vi "ArmControlCalibrate.vi"() -> ()   [LabVIEW 2014]
uses:
  <vilib>/Rock Robotics/WPI/CAN/TalonSRX/WPI_CANTalonSRX_APIFeedbackSelect.ctl
  <vilib>/Rock Robotics/WPI/Joystick/WPI_JoystickDeviceEnum.ctl
  <vilib>/Rock Robotics/WPI/CAN/TalonSRX/WPI_CANTalonSRX_APIControlMode.ctl
  <vilib>/Platform/TimedLoop/XDataNode/timing_clust.ctl
  <vilib>/Platform/TimedLoop/XDataNode/nitl_modes.ctl
  <vilib>/Platform/TimedLoop/XDataNode/wakeup.ctl
  <vilib>/Rock Robotics/WPI/SafetyOutput/WPI_SafetyOutputConfigMenu.ctl
  <vilib>/Rock Robotics/WPI/MotorControl/WPI_MotorControlOpenCANTalonSRX.vi
  Team900-VIs/Logitech/F510/F510-X.vi
  <vilib>/Utility/config.llb/Write Key (Double).vi
  <vilib>/Platform/TimedLoop/XDataNode/XDataNode.xnode
  <vilib>/Platform/TimedLoop/XDataNode/XDNodeRunTimeDep.lvlib
  <vilib>/Utility/config.llb/NI_LVConfig.lvlib
panel:
  in  "Motor to set offset":enum16{"Pivot", "Wrist", "Claw"}(ring)
  in  "Set":bool
  in  "stop":bool
  in  "Mode":enum32{"Manual Mode", "PID Tuning"}(tab)
  out "(manual) error out":errorcluster
  out "Sensor Position":dbl
  in  "Control this motor":enum16{"Pivot", "Extension", "Wrist", "Claw"}(ring)
  in  "Max %Vbus":dbl=0.1 format="%#_13g"
  in  "Motor Controller":enum16{"Pivot", "Extension", "Wrist"}(ring)
  in  "PID":cluster{"P":dbl, "I":dbl, "D":dbl}
  out "error out":errorcluster
  in  "Set":bool=TRUE
  in  "Ramp Rate":dbl
  out "Applied Throttle":dbl
  out "Encoder Position":dbl
  out "Analog In":dbl
  out "Sensor Position":dbl
  in  "Enable":bool
  in  "Desired Distance (in) or Angle (rad)":dbl format="%#_13g"
  out "Difference":dbl
  out "Waveform Chart":T1(graph)
  in  "Wrist Offset":dbl format="%#_13g"
  in  "Extension Offset":dbl format="%#_13g"
  in  "Pivot Offset":dbl format="%#_13g"
  in  "Invert Motor (set this before opening)":bool
  # "360 Ticks on extension"
  # "Left Stick controls whatever motor is selected"
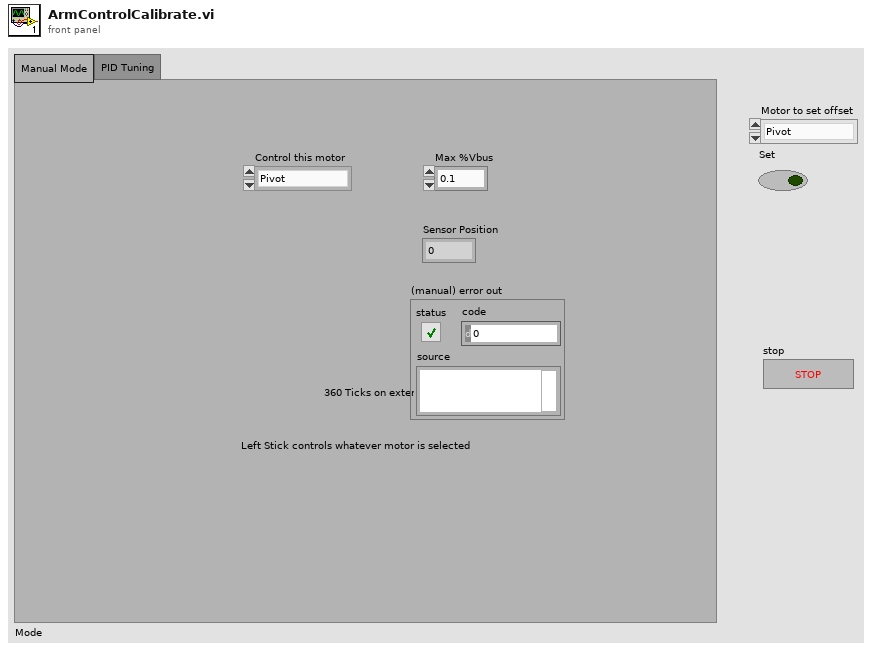
[diagram p1: front panel]
types:
  T1 = cluster{dbl, "Desired Distance (in) or Angle (rad)":dbl}
  T2 = typedef "NI_LVConfig.lvlib/Config Data RefNum.ctl" = refnum<k1>
  T3 = typedef "WPI_JoystickDeviceEnum.ctl" = enum16{"USB 0", "USB 1", "USB 2", "USB 3", "USB 4", "USB 5"}
  T4 = typedef "WPI_CANTalonSRX_APIControlMode.ctl" = enum8{"Percent VBus", "Speed", "Position", "Slave", "Unchanged / Invalid"}
  T5 = typedef "WPI_SafetyOutputConfigMenu.ctl" = enum16{"Enable", "Disable"}
  T6 = typedef "WPI_CANTalonSRX_APIFeedbackSelect.ctl" = enum16{"Digital Quadrature Encoder", "Analog Potentiometer", "Analog Encoder"}
  T7 = typedef "XDNodeRunTimeDep.lvlib/timing_clust.ctl" = cluster{"Expected End [f-1]":u64, "Actual End [f-1]":u64, "Finished Late? [f-1]":bool, "Expected End [i-1]":u64, "Actual End [i-1]":u64, "Finished Late? [i-1]":bool, "Expected Start [i]":u64, "Actual Start [i]":u64, "Expected Start [f]":u64, "Actual Start [f]":u64, "Source Name":string, "Structure Name":string, "Period":i64, "Deadline":i64, "Offset":i64, "Start":i64, "Priority":i32, "Timeout":i32, "Mode":T8, "Wakeup Reason":T9, "Error":errorcluster, "Source Type":string, "Secondary Source Type":string, "Global End Time":u64, "Global Start Time":u64, "Frame Duration":u64, "Iteration Duration":u64, "Assigned CPU":i32, "I/O Scan Engine Mode":u32}
  T8 = typedef "XDNodeRunTimeDep.lvlib/nitl_modes.ctl" = enum32{"No Change", "Process missed periods, maintain original phase", "Discard missed periods, maintain original phase", "Process missed periods, ignore original phase", "Discard missed periods, ignore original phase"}
  T9 = typedef "XDNodeRunTimeDep.lvlib/wakeup.ctl" = enum32{"Normal", "Aborted", "Asynchronous wakeup", "Timing source error", "Timed loop error", "Timeout"}
  T10 = typedef "WPI_MotorControlDeviceRef.ctl" = cluster{"DeviceStatus":errorcluster, "Type":T11, "PWM":cluster{"Controller":T12, "PWM Channel":T13, "DeadBand":T14}, "CAN":cluster{"Device Number":u8, "Control Mode":T15, "Semaphore":T16, "Max Vout":dbl, "TalonSRX Control Mode":T4}, "Invert":bool, "TransformRef":T17, "InvTransformRef":T17}
  T11 = typedef "WPI_MotorControlType.ctl" = enum16{"PWM", "CAN", "CANTalonSRX"}
  T12 = typedef "FPGA_TypedefDigitalModule.ctl" = enum16{"Controller 1"}
  T13 = typedef "FPGA_DIOPWMChannel.ctl" = enum8{"PWM 0", "PWM 1", "PWM 2", "PWM 3", "PWM 4", "PWM 5", "PWM 6", "PWM 7", "PWM 8", "PWM 9", "PWM MXP 0", "PWM MXP 1", "PWM MXP 2", "PWM MXP 3", "PWM MXP 4", "PWM MXP 5", "PWM MXP 6", "PWM MXP 7", "PWM MXP 8", "PWM MXP 9", "Invalid"}
  T14 = typedef "WPI_PWMDeadband.ctl" = cluster{"Name":string, "maxPositivePwm":i32, "minPositivePwm":i32, "centerPwm":i32, "maxNegativePwm":i32, "minNegativePwm":i32, "angularRange":u16}
  T15 = typedef "WPI_CANJaguar_ControlMode.ctl" = enum8{"Percent VBus", "Current", "Speed", "Position", "Voltage"}
  T16 = typedef "Semaphore RefNum" = refnum<k1>
  T17 = typedef "WPI_PWMTransform_ConPane.ctl" = refnum<vi>
  T18 = typedef "WPI_JoystickDevRef.ctl" = cluster{"Device":T3}
  T19 = typedef "WPI_CANTalonSRX_GlobalStatus.ctl" = cluster{"Applied Throttle":dbl, "Module Enabled":bool, "CAN Error":errorcluster, "Closed Loop Error":dbl, "Forward Limit Switch Closed":bool, "Reverse Limit Switch Closed":bool, "Sensor Position":dbl, "Sensor Velocity":dbl, "Current":dbl, "Sticky Fault - Over Temp":bool, "Sticky Fault - Under Voltage":bool, "Sticky Fault - Forward Limit":bool, "Sticky Fault - Reverse Limit":bool, "Sticky Fault - Forward Soft Limit":bool, "Sticky Fault - Reverse Soft Limit":bool, "Brake is Enabled":bool, "Encoder Position":dbl, "Encoder Velocity":dbl, "Encoder Index Count":dbl, "Encoder A Pin State":bool, "Encoder B Pin State":bool, "Encoder Index Pin State":bool, "Analog In":dbl, "Analog In Velocity":dbl, "Temperature (C)":dbl, "Battery Voltage":dbl}
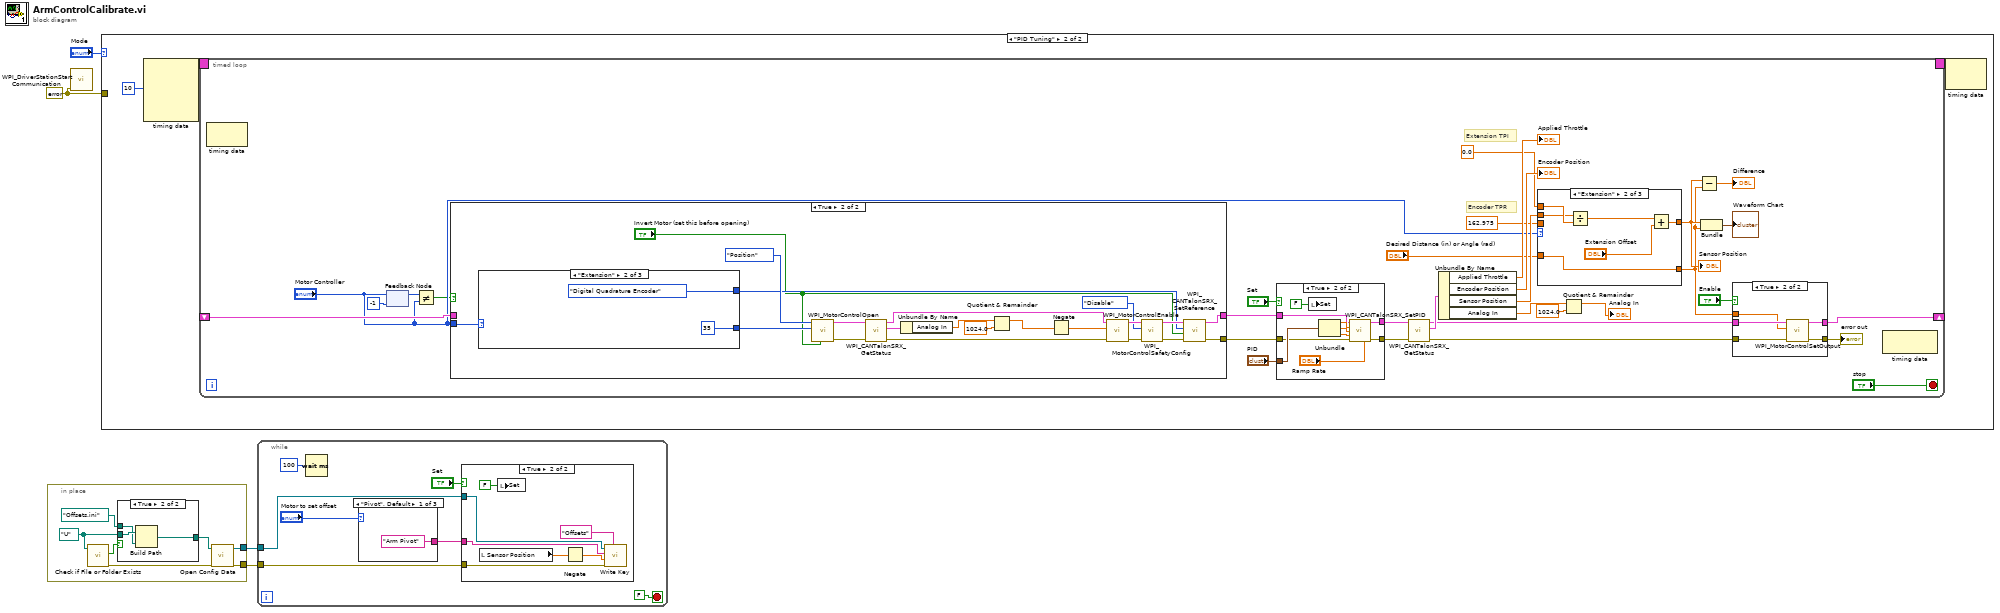
[diagram p0: block diagram]
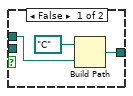
[diagram p2: hidden frame]
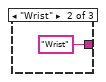
[diagram p3: hidden frame]
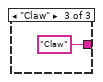
[diagram p4: hidden frame]
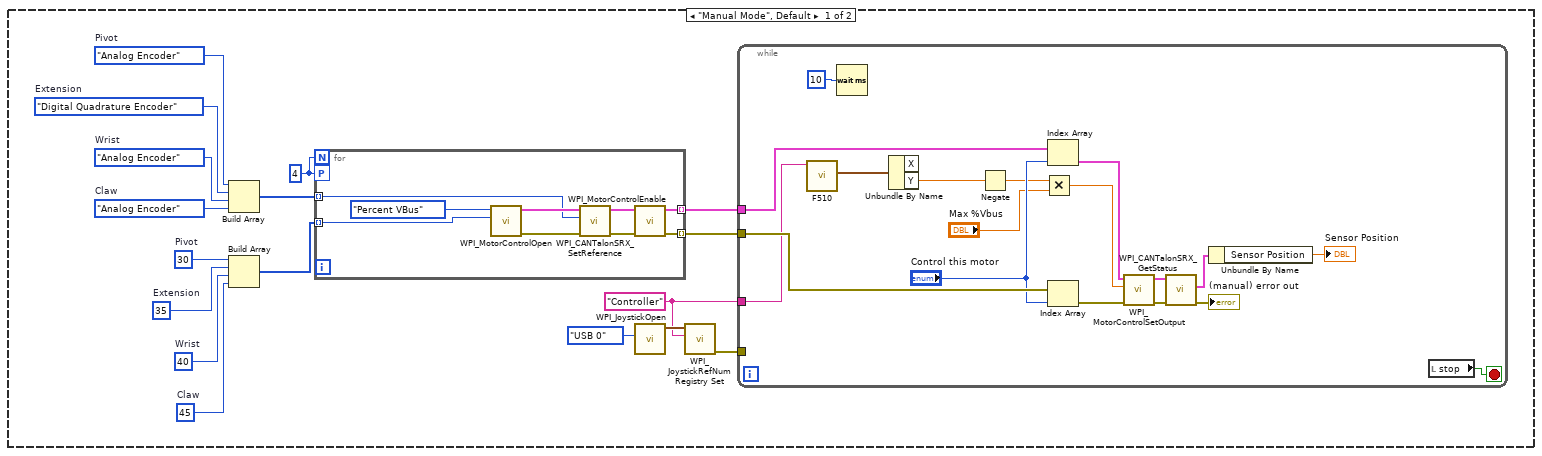
[diagram p6: hidden frame]
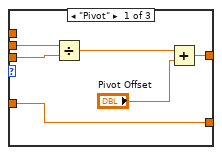
[diagram p7: hidden frame]
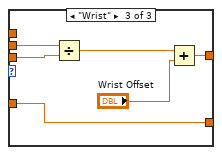
[diagram p8: hidden frame]
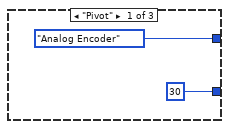
[diagram p10: hidden frame]
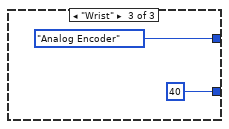
[diagram p11: hidden frame]
diagram:
  w3 = errorcluster {"status"=FALSE, "code"=0, "source"=""} ("error constant")
  n1 = in-place {
    in-place-border: [w10] -> w2
    in-place-border: [w9] -> w1
    w5 = path "U:/" ("base path")
    n2 = call <vilib>:"Check if File or Folder Exists.vi"("path"=w5) -> ("error out"=w11:errorcluster, "file or folder exists?"=w6:bool)  [unwired: 8 in, 1 out]
    n3 = case shown="True" w6 {
      tunnel: path "Offsets.ini" ("default name") -> [w14 w15]
      tunnel: [w13 w16] -> w8
      tunnel: w5 -> [_ w17]
      frame False {
        n4 = Build Path(base path=path "C:/", name or relative path=w14) -> (appended path=w13:path)
      }
      frame True {
        n5 = Build Path(base path=w17, name or relative path=w15) -> (appended path=w16:path)
      }
    }
    n6 = call <vilib>:"Open Config Data.vi"("error in (no error)"=w11, "configuration file path"=w8) -> ("error out"=w10:errorcluster, "refnum"=w9:T2)  [unwired: 1 in, 7 out]
  }
  n7 = call <vilib>:"WPI_DriverStationStart Communication.vi"("error in (no error)"=w3) -> ()  [unwired: 11 in]
  n8 = case shown="\"PID Tuning\"" "Mode" {
    tunnel: w3 -> [_ _]
    frame "Manual Mode", Default {
      w18 = u8 45  # Claw
      w19 = WPI_CANTalonSRX_APIFeedbackSelect."Analog Encoder"  # Claw
      w21 = "Controller" ("refnum name")
      w24 = WPI_CANTalonSRX_APIFeedbackSelect."Analog Encoder"  # Wrist
      w25 = WPI_CANTalonSRX_APIFeedbackSelect."Analog Encoder"  # Pivot
      w26 = WPI_CANTalonSRX_APIFeedbackSelect."Digital Quadrature Encoder"  # Extension
      w30 = u8 40  # Wrist
      w31 = u8 35  # Extension
      w32 = u8 30  # Pivot
      w34 = 4
      n9 = Build Array(w25, w26, w24, w19) -> (w27:T6[])
      n10 = Build Array(w32, w31, w30, w18) -> (w33:u8[])
      n11 = for {
        N: w34 -> [_]
        workers-P: w34 -> [_]
        tunnel: w33 -> [w61] mode=indexing
        tunnel: [w60] -> w29 mode=indexing
        tunnel: [w59] -> w28 mode=indexing
        tunnel: w27 -> [w53] mode=indexing
        n12 = call-poly <vilib>:"WPI_MotorControlOpen.vi"("Device Number"=w61, "Control Mode"=WPI_CANTalonSRX_APIControlMode."Percent VBus") -> ("error out"=w57:errorcluster, "MotorControlDeviceRef"=w56:T10)  [unwired: 8 in]
        n13 = call <vilib>:"WPI_CANTalonSRX_SetReference.vi"("error in (no error)"=w57, "Feedback Reference"=w53, "CAN Talon SRX Ref"=w56) -> ("error out"=w54:errorcluster, "CAN Talon SRX Ref Out"=w55:T10)  [unwired: 7 in]
        n14 = call <vilib>:"WPI_MotorControlEnable.vi"("error in (no error)"=w54, "CAN Jaguar Ref"=w55) -> ("error out"=w59:errorcluster, "CAN Jaguar Ref Out"=w60:T10)  [unwired: 8 in]
      }
      n15 = call <vilib>:"WPI_JoystickOpen.vi"("JoystickDevice"=WPI_JoystickDeviceEnum."USB 0") -> ("JoystickDevRef"=w23:T18)  [unwired: 10 in]
      n16 = call <vilib>:"WPI_JoystickRefNum Registry Set.vi"("refnum name"=w21, "JoystickDevRef"=w23) -> ("error out"=w20:errorcluster)  [unwired: 8 in, 1 out]
      n17 = while {
        tunnel: w29 -> [w51]
        tunnel: w28 -> [w50]
        tunnel: w21 -> [w48]
        tunnel: w20 -> [_]
        stop <- w41 stop-if-true
        n18 = call-poly "F510.vi"("refnum name"=w48) -> ("Left Stick"=w45:cluster{"X":dbl, "Y":dbl})  [unwired: 4 in, 6 out]
        n19 = Wait (ms)(milliseconds to wait=u32 10) -> ()  [unwired: 1 out]
        n20 = Unbundle By Name(w45) -> ("Y"=w44:dbl)  [unwired: 1 out]
        n21 = Negate(x=w44) -> (-x=w35:dbl)
        n22 = Multiply(x=w35, y="Max %Vbus") -> (x*y=w42:dbl)
        n23 = Index Array(array=w51, index="Control this motor") -> (element=w37:T10)
        n24 = Index Array(array=w50, index="Control this motor") -> (element=w36:errorcluster)
        n25 = call <vilib>:"WPI_MotorControlSetOutput.vi"("error in (no error)"=w36, "Output"=w42, "MotorControlDevRef"=w37) -> ("error out"=w40:errorcluster, "MotorControlDevRef"=w39:T10)  [unwired: 6 in, 1 out]
        n26 = call <vilib>:"WPI_CANTalonSRX_GetStatus.vi"("error in (no error)"=w40, "CAN Talon SRX Ref"=w39) -> ("error out"=→"(manual) error out":errorcluster, "Talon SRX Status"=w38:T19)  [unwired: 7 in, 1 out]
        n27 = Unbundle By Name(w38) -> ("Sensor Position"=→"Sensor Position":dbl)
        n28 = local read "stop"() -> (w41:bool)
      }
    }
    frame "PID Tuning" {
      n29 = node-c288(i64 10 ("Period")) -> (w64:T7)  [unwired: 3 in]
      n30 = timed-loop {
        timing: w64 -> [_]
        timing-out: [_] -> w63
        shift-right: [w74] -> _
        shift-left: _ -> [w75]
        stop <- "stop" stop-if-true
        # "Extension TPI"
        # "Encoder TPR"
        n31 = node-c288() -> ()  [unwired: 1 in, 1 out]
        n32 = feedback #1(-1) -> (w94:i32)
        n33 = feedback-in #1("Motor Controller") -> ()
        n34 = Not Equal?(x=w94, y="Motor Controller") -> (x != y?=w69:bool)
        n35 = case shown="True" w69 {
          tunnel: [w114 w133] -> w90
          tunnel: [_ w132] -> w85
          tunnel: "Motor Controller" -> [_ w116]
          tunnel: w75 -> [w114 _]
          frame False {
          }
          frame True {
            n36 = case shown="\"Extension\"" w116 {
              tunnel: [u8 30 ("Device Number") u8 35 ("Device Number") u8 40 ("Device Number")] -> w134
              tunnel: [WPI_CANTalonSRX_APIFeedbackSelect."Analog Encoder" ("Feedback Reference") WPI_CANTalonSRX_APIFeedbackSelect."Digital Quadrature Encoder" ("Feedback Reference") WPI_CANTalonSRX_APIFeedbackSelect."Analog Encoder" ("Feedback Reference")] -> w121
              frame "Pivot" {
              }
              frame "Extension" {
              }
              frame "Wrist" {
              }
            }
            n37 = call-poly <vilib>:"WPI_MotorControlOpen.vi"("Invert"="Invert Motor (set this before opening)", "Device Number"=w134, "Control Mode"=WPI_CANTalonSRX_APIControlMode."Position") -> ("error out"=w120:errorcluster, "MotorControlDeviceRef"=w131:T10)  [unwired: 7 in]
            n38 = call <vilib>:"WPI_CANTalonSRX_GetStatus.vi"("error in (no error)"=w120, "CAN Talon SRX Ref"=w131) -> ("error out"=w119:errorcluster, "Talon SRX Status"=w130:T19, "CAN Talon SRX Ref Out"=w127:T10)  [unwired: 7 in]
            n39 = Unbundle By Name(w130) -> ("Analog In"=w126:dbl)
            n40 = Quotient & Remainder(x=w126, y=1024.0) -> (x-y*floor(x/y)=w124:dbl)  [unwired: 1 out]
            n41 = Negate(x=w124) -> (-x=w123:dbl)
            n42 = call <vilib>:"WPI_MotorControlEnable.vi"("error in (no error)"=w119, "Encoder Initial Position"=w123, "CAN Jaguar Ref"=w127) -> ("error out"=w118:errorcluster, "CAN Jaguar Ref Out"=w128:T10)  [unwired: 7 in]
            n43 = call <vilib>:"WPI_MotorControlSafetyConfig.vi"("error in (no error)"=w118, "mode"=WPI_SafetyOutputConfigMenu."Disable", "MotorControlDevRef"=w128) -> ("error out"=w117:errorcluster, "MotorControlDevRef"=w129:T10)  [unwired: 7 in]
            n44 = call <vilib>:"WPI_CANTalonSRX_SetReference.vi"("error in (no error)"=w117, "Reverse Feedback Sensor"="Invert Motor (set this before opening)", "Feedback Reference"=w121, "CAN Talon SRX Ref"=w129) -> ("error out"=w132:errorcluster, "CAN Talon SRX Ref Out"=w133:T10)  [unwired: 6 in]
          }
        }
        n45 = case shown="True" "Set" {
          tunnel: "PID" -> [_ w157]
          tunnel: w90 -> [w149 w156]
          tunnel: [w149 w154] -> w89
          tunnel: [w150 w153] -> w87
          tunnel: w85 -> [w150 w152]
          frame False {
          }
          frame True {
            n46 = local write "Set"(FALSE) -> ()
            n47 = Unbundle(w157) -> ("P"=w158:dbl, "I"=w159:dbl, "D"=w160:dbl)
            n48 = call <vilib>:"WPI_CANTalonSRX_SetPID.vi"("CAN Talon SRX Ref"=w156, "P"=w158, "I"=w159, "D"=w160, "error in (no error)"=w152, "Ramp Rate"="Ramp Rate") -> ("CAN Talon SRX Ref Out"=w154:T10, "error out"=w153:errorcluster)  [unwired: 8 in]
          }
        }
        n49 = call <vilib>:"WPI_CANTalonSRX_GetStatus.vi"("error in (no error)"=w87, "CAN Talon SRX Ref"=w89) -> ("error out"=w78:errorcluster, "Talon SRX Status"=w88:T19, "CAN Talon SRX Ref Out"=w79:T10)  [unwired: 7 in]
        n50 = Unbundle By Name(w88) -> ("Applied Throttle"=→"Applied Throttle":dbl, "Encoder Position"=→"Encoder Position":dbl, "Sensor Position"=w73:dbl, "Analog In"=w83:dbl)
        n51 = case shown="\"Extension\"" "Motor Controller" {
          tunnel: w73 -> [w98 w106 w112]
          tunnel: 162.975 ("TPR") -> [w97 _ w113]
          tunnel: [w99 w103 w109] -> w67
          tunnel: 0.0 ("Extension TPI") -> [_ w107 _]
          tunnel: [w96 w105 w108] -> w66
          tunnel: "Desired Distance (in) or Angle (rad)" -> [w96 w105 w108]
          frame "Pivot" {
            n52 = Divide(x=w98, y=w97) -> (x/y=w101:dbl)
            n53 = Add(x=w101, y="Pivot Offset") -> (x+y=w99:dbl)
          }
          frame "Extension" {
            n54 = Divide(x=w106, y=w107) -> (x/y=w102:dbl)
            n55 = Add(x=w102, y="Extension Offset") -> (x+y=w103:dbl)
          }
          frame "Wrist" {
            n56 = Divide(x=w112, y=w113) -> (x/y=w110:dbl)
            n57 = Add(x=w110, y="Wrist Offset") -> (x+y=w109:dbl)
          }
        }
        "Sensor Position" <- w67
        n58 = Quotient & Remainder(x=w83, y=1024.0) -> (x-y*floor(x/y)=→"Analog In":dbl)  [unwired: 1 out]
        n59 = Subtract(x=w67, y=w66) -> (x-y=→"Difference":dbl)
        n60 = Bundle(w67, "Desired Distance (in) or Angle (rad)"=w66) -> (→"Waveform Chart":T1)  [unwired: 1 in]
        n61 = case shown="True" "Enable" {
          tunnel: w79 -> [w142 w148]
          tunnel: w78 -> [w143 w147]
          tunnel: [w143 w146] -> w95
          tunnel: [w142 w145] -> w74
          tunnel: w66 -> [_ w144]
          frame False {
          }
          frame True {
            n62 = call <vilib>:"WPI_MotorControlSetOutput.vi"("error in (no error)"=w147, "Output"=w144, "MotorControlDevRef"=w148) -> ("error out"=w146:errorcluster, "MotorControlDevRef"=w145:T10)  [unwired: 6 in, 1 out]
          }
        }
        "error out" <- w95
        n63 = node-c288() -> ()  [unwired: 1 in, 1 out]
      }
      n64 = node-c288(w63) -> ()  [unwired: 1 out]
    }
  }
  n65 = while {
    tunnel: w2 -> [w172]
    tunnel: w1 -> [w173]
    stop <- FALSE stop-if-true
    n66 = Wait (ms)(milliseconds to wait=u32 100) -> ()  [unwired: 1 out]
    n67 = case shown="\"Pivot\", Default" "Motor to set offset" {
      tunnel: ["Arm Pivot" "Wrist" "Claw"] -> w167
      frame "Pivot", Default {
      }
      frame "Wrist" {
      }
      frame "Claw" {
      }
    }
    n68 = case shown="True" "Set" {
      tunnel: w173 -> [_ w182]
      tunnel: w172 -> [_ w181]
      tunnel: w167 -> [_ w177]
      frame False {
      }
      frame True {
        n69 = local read "Sensor Position"() -> (w180:dbl)
        n70 = local write "Set"(FALSE ("Zero Position")) -> ()
        n71 = Negate(x=w180) -> (-x=w179:dbl)
        n72 = call-poly <vilib>:"Write Key.vi"("section"="Offsets", "error in (no error)"=w181, "value"=w179, "key"=w177, "refnum"=w182) -> ()  [unwired: 4 in, 3 out]
      }
    }
  }
